vi "读取信息.vi"(8 "error in (no error)":errorcluster caption="错误输入（无错误）") -> (0 "error out":errorcluster caption="错误输出", 3 "输出信息":string)   [LabVIEW 2011, in "单例.lvlib"]
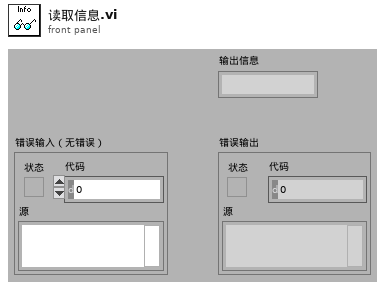
[diagram p1: front panel]
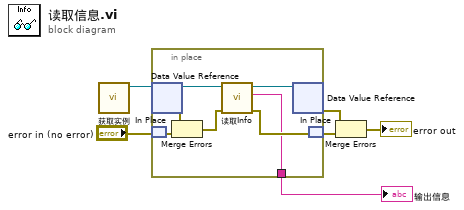
[diagram p0: block diagram]
diagram:
  n1 = call "获取实例.vi"() -> ("data value reference"=w6:refnum<data-value>)  [unwired: 11 in]
  n2 = in-place {
    in-place-border: [w7] -> w1
    n3 = in-place-dvr #1(w6) -> (w11:refnum<class "单例.lvclass">, w13:errorcluster)
    n4 = in-place-match #2("error in (no error)") -> (w12:errorcluster)
    n5 = Merge Errors(w13, w12) -> (w9:errorcluster)
    n6 = call "读取Info.vi"("error in (no error)"=w9, "单例输入"=w11) -> ("error out"=w8:errorcluster, "Info"=w7:string, "单例输出"=w10:refnum<class "单例.lvclass">)  [unwired: 7 in]
    n7 = in-place-dvr #1(w10) -> (w3:errorcluster)  [unwired: 1 out]
    n8 = in-place-match #2(w8) -> (w4:errorcluster)
  }
  "输出信息" <- w1
  n9 = Merge Errors(w3, w4) -> (→"error out":errorcluster)
